vi "Debug_FilterTable.vi"(9 "QueuesToDisplay":string[](array[string]), 10 "MessagesToDisplay":string[](array[string]), 11 "Array in":string[][](array[string])) -> (3 "Array out":string[][](array[string]))   [LabVIEW 2017, in "Server.lvlib" / "Message Queue.lvlib"]
uses:
  Message Queue.lvlib
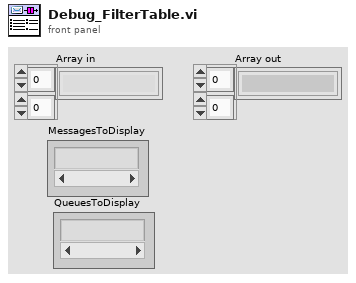
[diagram p1: front panel]
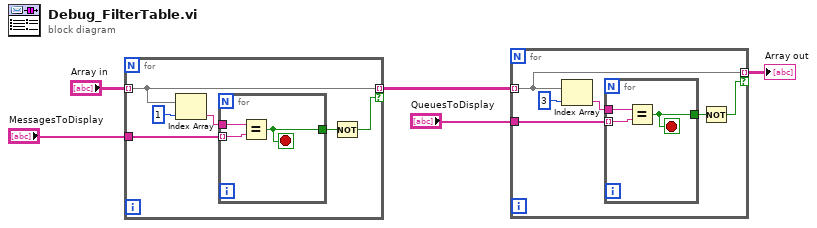
[diagram p0: block diagram]
diagram:
  n1 = for {
    tunnel: "Array in" -> [w8] mode=indexing
    tunnel: "MessagesToDisplay" -> [w10]
    tunnel: [w8] -> w3 mode=indexing if=w6
    n2 = Index Array(array=w8, index=1) -> (element=w9:string)
    n3 = for {
      tunnel: w10 -> [w13] mode=indexing
      tunnel: w9 -> [w14]
      tunnel: [w12] -> w7
      stop <- w12 stop-if-true
      n4 = Equal?(x=w14, y=w13) -> (x = y?=w12:bool)
    }
    n5 = Not(x=w7) -> (.not. x?=w6:bool)
  }
  n6 = for {
    tunnel: w3 -> [w17] mode=indexing
    tunnel: "QueuesToDisplay" -> [w19]
    tunnel: [w17] -> w1 mode=indexing if=w15
    n7 = Index Array(array=w17, index=3) -> (element=w18:string)
    n8 = for {
      tunnel: w19 -> [w22] mode=indexing
      tunnel: w18 -> [w23]
      tunnel: [w21] -> w16
      stop <- w21 stop-if-true
      n9 = Equal?(x=w23, y=w22) -> (x = y?=w21:bool)
    }
    n10 = Not(x=w16) -> (.not. x?=w15:bool)
  }
  "Array out" <- w1
